vi "GUI_Single Button Pump.vi"() -> ()   [LabVIEW 2011] (continued)
        w2202 = T33[] [enum."EXIT GPM Mode LB", enum."EXIT GPM Mode EC"] items=["No Action", "Set GPM Mode LB", "EXIT GPM Mode LB", "Set GPM Mode EC", "EXIT GPM Mode EC", "Set GVM mode LB", "Set GVM Mode EC", "Open LB Backing Valve", "Open EC Backing Valve", "Open EC Roughing Valve", "Open LB Roughing Valve", "Open M123 Roughing Valve", "Close M123 Roughing Valve", "Open Compressor Roughing Valve", "Close Compressor Roughing Valve", "Open BeamDump Roughing Valve", "Close BeamDump Roughing Valve", "Open OAP Roughing Valve", "Close OAP Roughing Valve", "Open BTL Roughing Valve", "Close BTL Roughing Valve", "Open Target Roughing Valve", "Close Target Roughing Valve", "Open BTL2 Roughing Valve", "Close BTL2 Roughing Valve", "Open HPD Roughing Valve", "Close HPD Roughing Valve", "LB Start Roughing Pump ", "EC Start Roughing Pump", "Open COMP Turbo Backing Valve", "Open M123 Turbo Backing Valve", "Open OAP Turbo Backing Valve", "Open HPBD Turbo Backing Valve", "Open BLT Turbo Backing Valve", "Open TARGET1 Turbo Backing Valve", "Open TARGET2 Turbo Backing Valve", "Open BLT2 Turbo Backing Valve", "Open HPD Turbo Backing Valve", "LB Start Turbo Backing Pump", "EC Start Turbo Backing Pump", "Start COMP Turbo Pump", "Start M123 Turbo Pump", "Start OAP Turbo Pump", "Start BTL Turbo Pump", "Start TARGET1 Turbo Pump", "Start TARGET2 Turbo Pump", "Start BTL2 Turbo Pump", "Start HPD Turbo Pump", "Open COMP Turbo Gate Valve", "Open M123 Turbo Gate Valve", "Open OAP Turbo Gate Valve", "Open BTL Turbo Gate Valve", "Open TARGET1 Turbo Gate Valve", "Open TARGET2 Turbo Gate Valve", "Open BTL2 Turbo Gate Valve", "Open HPD Turbo Gate Valve"]
        # "Open Backing Valves on both systems"
        n866 = Unbundle By Name(w2204) -> ("TCPConnection.Command TCP Connection EC"=w2211:refnum<k5>)
        n867 = Unbundle By Name(w2204) -> ("TCPConnection.Command TCP Connection LB"=w2213:refnum<k5>)
        n868 = call "Build Command.vi"("Command Array in"=w2202, "input cluster"=w2204) -> ("output EC Command cluster"=w2212:T34, "output LB Command cluster"=w2214:T34)  [unwired: 8 in]
        n869 = call "Send Command LB.vi"("error in (no error)"=w2210, "output LB Command cluster"=w2214, "TCP Network Connection in"=w2213) -> ("error out"=w2208:errorcluster)  [unwired: 8 in]
        n870 = call "Send Command EC.vi"("error in (no error)"=w2210, "output EC Command cluster"=w2212, "TCP Network Connection in"=w2211) -> ("error out"=w2209:errorcluster)  [unwired: 8 in]
        n871 = Merge Errors(w2208, w2209) -> (w2206:errorcluster)
        n872 = call "Reset Command Clusters.vi"("error in (no error)"=w2206, "input cluster"=w2204) -> ("error out"=w2205:errorcluster, "output cluster"=w2203:T20)  [unwired: 8 in]
        n873 = call <vilib>:"Add State(s) to Queue__jki_lib_state_machine.vi"("State(s) in Front (\"\")"="Main: Check GPM GVM Mode Status>>end", "State(s) in (\"\")"=w2216) -> ("States Out"=w2215:string)  [unwired: 13 in]
      }
      frame "Main: Open Turbo Gate Valves" {
        w2218 = T33[] [enum."Open M123 Turbo Gate Valve", enum."Open OAP Turbo Gate Valve", enum."Open BTL Turbo Gate Valve", enum."Open TARGET1 Turbo Gate Valve", enum."Open TARGET2 Turbo Gate Valve", enum."Open BTL2 Turbo Gate Valve", enum."Open HPD Turbo Gate Valve"] items=["No Action", "Set GPM Mode LB", "EXIT GPM Mode LB", "Set GPM Mode EC", "EXIT GPM Mode EC", "Set GVM mode LB", "Set GVM Mode EC", "Open LB Backing Valve", "Open EC Backing Valve", "Open EC Roughing Valve", "Open LB Roughing Valve", "Open M123 Roughing Valve", "Close M123 Roughing Valve", "Open Compressor Roughing Valve", "Close Compressor Roughing Valve", "Open BeamDump Roughing Valve", "Close BeamDump Roughing Valve", "Open OAP Roughing Valve", "Close OAP Roughing Valve", "Open BTL Roughing Valve", "Close BTL Roughing Valve", "Open Target Roughing Valve", "Close Target Roughing Valve", "Open BTL2 Roughing Valve", "Close BTL2 Roughing Valve", "Open HPD Roughing Valve", "Close HPD Roughing Valve", "LB Start Roughing Pump ", "EC Start Roughing Pump", "Open COMP Turbo Backing Valve", "Open M123 Turbo Backing Valve", "Open OAP Turbo Backing Valve", "Open HPBD Turbo Backing Valve", "Open BLT Turbo Backing Valve", "Open TARGET1 Turbo Backing Valve", "Open TARGET2 Turbo Backing Valve", "Open BLT2 Turbo Backing Valve", "Open HPD Turbo Backing Valve", "LB Start Turbo Backing Pump", "EC Start Turbo Backing Pump", "Start COMP Turbo Pump", "Start M123 Turbo Pump", "Start OAP Turbo Pump", "Start BTL Turbo Pump", "Start TARGET1 Turbo Pump", "Start TARGET2 Turbo Pump", "Start BTL2 Turbo Pump", "Start HPD Turbo Pump", "Open COMP Turbo Gate Valve", "Open M123 Turbo Gate Valve", "Open OAP Turbo Gate Valve", "Open BTL Turbo Gate Valve", "Open TARGET1 Turbo Gate Valve", "Open TARGET2 Turbo Gate Valve", "Open BTL2 Turbo Gate Valve", "Open HPD Turbo Gate Valve"]
        # "Event TAG"
        # "Check if Open first"
        # "Open Backing Valves on both systems"
        n874 = Unbundle By Name(w2221) -> ("TCPConnection.Command TCP Connection LB"=w2230:refnum<k5>)
        n875 = Unbundle By Name(w2221) -> ("TCPConnection.Command TCP Connection EC"=w2228:refnum<k5>)
        n876 = call "Build Command.vi"("Command Array in"=w2218, "input cluster"=w2221) -> ("output EC Command cluster"=w2229:T34, "output LB Command cluster"=w2231:T34)  [unwired: 8 in]
        n877 = call "Send Command LB.vi"("error in (no error)"=w2227, "output LB Command cluster"=w2231, "TCP Network Connection in"=w2230) -> ("error out"=w2225:errorcluster)  [unwired: 8 in]
        n878 = call "Send Command EC.vi"("error in (no error)"=w2227, "output EC Command cluster"=w2229, "TCP Network Connection in"=w2228) -> ("error out"=w2226:errorcluster)  [unwired: 8 in]
        n879 = Merge Errors(w2225, w2226) -> (w2224:errorcluster)
        n880 = call "Reset Command Clusters.vi"("error in (no error)"=w2224, "input cluster"=w2221) -> ("error out"=w2223:errorcluster, "output cluster"=w2222:T20)  [unwired: 8 in]
        n881 = call "MID-VAC Timer.vi"("TO sec (Start timer)"=5.0, "Action"=timerAction_typdef."Start Timer") -> ()  [unwired: 9 in, 1 out]
        n882 = call <vilib>:"Add State(s) to Queue__jki_lib_state_machine.vi"("State(s) in Front (\"\")"="Main: Check Turbo Valve Status", "State(s) in (\"\")"=w2233) -> ("States Out"=w2232:string)  [unwired: 13 in]
      }
      frame "Main: Check Turbo Valve Status" {
        w2234 = T32[] [enum."Is M123 Turbo Gate Valve Opened? ", enum."Is OAP Turbo Gate Valve Opened?", enum."Is BTLTurbo Gate Valve Opened?", enum."Is TARGET Turbo Gate Valve 1Opened?", enum."Is TARGET Turbo Gate Valve 2 Opened?", enum."Is BTL2 Turbo Gate Valve Opened?", enum."Is HPD Turbo Gate Valve Opened?"] items=["No Action", "Is EC GPM Mode ON?", "Is EC GPM Mode Off?", "Is EC GVM Mode ON?", "Is EC GVM Off?", "Is  EC GPM or GVM Mode ON?", "Is LB GPM Mode ON?", "Is LB GPM Mode Off?", "Is LB GVM Mode ON?", "Is LB GVM Mode Off?", "Is  LB GPM or GVM Mode ON?", "Is M123 Turbo Gate Valve Opened? ", "Is M123 Turbo Gate Valve Closed?", "Is OAP Turbo Gate Valve Opened?", "Is OAP Turbo Gate Valve Closed?", "Is BTLTurbo Gate Valve Opened?", "Is BTL Turbo Gate Valve Closed?", "Is TARGET Turbo Gate Valve 1Opened?", "Is TARGET1 Turbo Gate Valve Closed?", "Is TARGET Turbo Gate Valve 2 Opened?", "Is TAREGT2 Turbo Gate Valve Closed?", "Is BTL2 Turbo Gate Valve Opened?", "Is BTL2 Turbo Gate Valve Closed?", "Is HPD Turbo Gate Valve Opened?", "Is HPD Turbo Gate Valve Closed?", "Is COMP to M123 gate Valve Opened?", "Is COMP to M123 Valve Closed?", "Is HPBD Gate Valve Opened?", "Is HPBD Gate Valve Closed?", "Is M123 to OAP gate valve opened?", "Is M123 to OAP gate valve closed?", "Is OAP to BLT gate valve opened?", "Is OAP to BTL Gate Valve Closed?", "Is BLT to TARGET gate valve opened?", "Is BTL to TARGET Gate Valve Closed?", "Is TARGET to BLT2 gate valve opened?", "Is TARGET to BTL2 Gate Valve Closed?", "Is BLT2 to HPD gate valve opened?", "Is BTL2 to HPD Gate Valve Closed?", "Is COMP at Atmospheric Pressure?", "Is M123 at Atmospheric Pressure?", "Is BeamDump at Atmospheric Pressure?", "Is OAP at Atmospheric Pressure?", "Is BLT at Atmospheric Pressure", "Is TARGET at Atmospheric Pressure?", "Is BLT2 at Atmospheric Pressure?", "Is HPD at Atmospheric Pressure?", "Is the EC Roughing Pump ON?", "Is the EC Roughing Pump OFF?", "Does the EC Roughing Pump have a fault?", "Is the LB Roughing Pump ON?", "Is the LB Roughing Pump Off?", "Does the LB Roughing Pump have a fault?", "Is the EC Backing Pump ON?", "Is the EC Backing Pump OFF?", "Is the LB Backing Pump ON?", "Is the LB Backing Pump OFF?", "Does the EC Backing Pump have a fault?", "Does the LB Backing Pump have a fault?", "Is the EC Backing Pipe at Atmospheric Pressure", "Is the LB Backing Pipe at Atmospheric Pressure", "Is the EC Backing Manifold at Atmospheric Pressure", "s the LB Backing Manifold at Atmospheric Pressure?", "Is the EC Roughing Pipe at Atmospheric Pressure", "Is the LB Roughing Pipe at Atmospheric Pressure?", "Is the EC Roughing Manifold at Atmospheric Pressure", "Is the LB Roughing Manifold at Atmospheric Pressure", "Is LB Backing Manifold Valve Opened?", "Is EC Backing Manifold Valve Opened?", "Is LB Roughing Manifold Valve Opened?", "Is EC Roughing Manifold Valve Opened?", "Is COMP Roughing Valve Opened?", "Is M123 Roughing Valve Opened?", "Is M123 Roughing Valve Closed?", "Is OAP Roughing Valve Opened?", "Is OAP Roughing Valve Closed?", "Is HPBD Roughing Valve Opened?", "Is HPBD Roughing Valve Closed?", "Is BTL Roughing Valve Opened?", "Is BTL Roughing Valve Closed?", "Is TARGET Roughing Valve Opened?", "Is TARGET Roughing Valve Closed?", "Is BTL2 Roughing Valve Opened?", "Is BTL2 Roughing Valve Closed?", "Is HPD Roughing Valve Opened?", "Is HPD Roughing Valve Closed?", "Is COMP Turbo Backing Valve Opened?", "Is M123 Turbo Backing Valve Opened", "Is HPBD Turbo Backing Valve Opened?", "Is OAP Turbo Backing Valve Opened?", "Is BTL Turbo Backing Valve Opened?", "Is TARGET1 Turbo Backing Valve Opened?", "Is TARGET2 Turbo Backing Valve Opened?", "Is BTL2 Turbo Backing Valve Opened?", "Is HPD Turbo Backing Valve Opened?", "Is M123 Backing at MID-VAC?", "Is OAP Backing at MID-VAC?", "Is TARGET1 Backing at MID-VAC?", "Is TARGET2 Backing at MID-VAC?", "Is BTL Backing at MID-VAC?", "Is BTL2 Backing at MID-VAC?", "Is HPD Backing at MID-VAC?", "Is M123 Turbo in Normal Operation", "Is COMP Turbo in Normal Operation", "Is OAP Turbo in Normal Operation", "Is BTL Turbo in Normal Operation", "Is TARGET1 Turbo in Normal Operation", "Is TARGET2 Turbo in Normal Operation", "Is BTL2 Turbo in Normal Operation", "Is HPD Turbo in Normal Operation", "Is M123 at MID-VAC?", "Is OAP at MID-VAC?", "Is COMP at MID-VAC?", "Is BTL at MID-VAC?", "Is TARGET at MID-VAC?", "Is BTL2 at MID-VAC?", "Is HPD at MID-VAC?"]
        w2247 = Error_codes."002-Turbo gate valve status" ("Error Codes")
        # "Check Conditions"
        # "Event TAG"
        n883 = call "GetAction.vi"("Check Condition"=w2247, "Query Array"=w2234, "input cluster"=w2237, "error in (no error)"=w2249) -> ("Status Array Out"=w2248:string[], "Generate Event?"=w2239:bool, "error out"=w2245:errorcluster)  [unwired: 6 in, 3 out]
        n884 = call "Generate User Event.vi"("Add(t)/Remove(f) Event"=w2239, "error in (no error)"=w2245, "User Event in"=w2246, "Status Array In"=w2248, "Error Codes"=w2247) -> ("error out"=w2244:errorcluster)  [unwired: 5 in, 1 out]
        n885 = Unbundle By Name(w2237) -> ("VI Refnum"=w2236:refnum<vi>)
        n886 = call "MID-VAC Timer.vi"("Action"=timerAction_typdef."Timer Running") -> ("TO"=w2242:bool)  [unwired: 10 in]
        n887 = Not A Number/Path/Refnum?(number/path/refnum=w2236) -> (NaN/Path/Refnum?=w2235:bool)
        n888 = And(x=w2239, y=w2242) -> (x .and. y?=w2241:bool)
        n889 = case shown="True" w2241 {
          tunnel: w2240 -> [_ w2282]
          frame False {
          }
          frame True {
            n890 = Bundle By Name(cluster=T14 {"vi path"=path "Dummy.vi", "Message"=""}, "vi path"=path "Two Button Screen" ("event data"), "Message"="Some Turbo Valves have not opened.\nClick on continue to wait for some more time.\nClick Exit to abort GPM" ("message")) -> (w2278:T14)
            n891 = Generate User Event(user event=w2282, event data cluster=w2278) -> ()  [unwired: 1 in, 2 out]
          }
        }
        n892 = case shown="True" w2239 {
          tunnel: ["next step" w2263] -> w2238
          tunnel: w2236 -> [w2252 w2262]
          tunnel: w2235 -> [w2253 w2261]
          frame False {
            n893 = case shown="True" w2253 {
              tunnel: w2252 -> [_ w2257]
              frame False {
              }
              frame True {
                n894 = invoke class="VI" method="Abort VI"(reference=w2257) -> (reference out=w2255:refnum<vi>, error out=w2256:errorcluster)  [unwired: 2 in, 1 out]
                n895 = case shown="No Error" w2256 {
                  selector: w2256 -> [w2259 _]
                  tunnel: w2255 -> [w2260 _]
                  frame No Error {
                    n896 = Close Reference(reference=w2260, error in (no error)=w2259) -> (error out=w2258:errorcluster)
                    n897 = invoke on="User Input Panel" class="SubPnl" method="Remove VI"(error in=w2258) -> ()  [unwired: 2 in, 3 out]
                  }
                  frame Error {
                  }
                }
              }
            }
          }
          frame True {
            # "when to is true\nand"
            n898 = case shown="False" w2261 {
              tunnel: w2262 -> [w2267 _]
              tunnel: [w2265 "Main: Check Chamber Pressures"] -> w2263
              frame False {
                n899 = call "FindControlByName_VEPS.vi"("control name"="Op Out", "vi refnum"=w2267) -> ("control refnum"=w2269:refnum<vi>)  [unwired: 2 in, 1 out]
                n900 = property class="Ctl"(reference=w2269) -> ("Value"=w2268:variant)  [unwired: 1 in, 2 out]
                n901 = Variant To Data(type=op_typdef."Idle" ("Op Out 3"), Variant=w2268) -> (data=w2266:T24)  [unwired: 1 in, 1 out]
                n902 = case shown="\"Ignore and Continue\"" w2266 {
                  tunnel: ["Main: Check Chamber Pressures" "Main: Check Turbo Valve Status" "Main: Final Display" "Idle\nMacro: Exit"] -> w2265
                  frame "Idle", Default {
                  }
                  frame "Continue to Wait" {
                    # "Continue to wait. Reset Timer"
                    n903 = call "MID-VAC Timer.vi"("TO sec (Start timer)"=30000.0, "Action"=timerAction_typdef."Start Timer") -> ()  [unwired: 9 in, 1 out]
                  }
                  frame "Ignore and Continue" {
                  }
                  frame "Exit" {
                  }
                }
              }
              frame True {
              }
            }
          }
        }
        n904 = call <vilib>:"Add State(s) to Queue__jki_lib_state_machine.vi"("State(s) in (\"\")"=w2251, "State(s) at Back (\"\")"=w2238) -> ("States Out"=w2250:string)  [unwired: 13 in]
      }
      frame "New Category: 2" {
        # "Your code here.\n(You can make a copy of, or modify, this frame)"
        n905 = call <vilib>:"Add State(s) to Queue__jki_lib_state_machine.vi"("State(s) in (\"\")"=w2286) -> ("States Out"=w2285:string)  [unwired: 14 in]
      }
    }
    n906 = case shown="True" w9 {
      tunnel: w11 -> [w25 w28]
      tunnel: [w25 w27] -> w10
      frame False {
      }
      frame True {
        n907 = call <vilib>:"Add State(s) to Queue__jki_lib_state_machine.vi"("State(s) in Front (\"\")"="Command: Get Status" ("State(s) in Front (\"\")"), "State(s) in (\"\")"=w28) -> ("States Out"=w27:string)  [unwired: 13 in]
      }
    }
  }
